vi "binary.vi"() -> ()   [LabVIEW 2020]
uses:
  <vilib>/Utility/error.llb/DialogType.ctl
panel:
  out "data":dbl[](array[numeric])
  out "Array":dbl[](array[numeric])
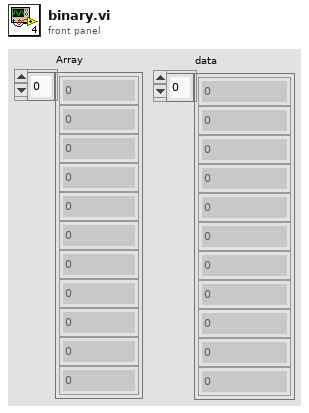
[diagram p1: front panel]
types:
  T1 = enum16{"open", "replace", "create", "open or create", "replace or create", "replace or create with confirmation"}
  T2 = typedef "DialogType.ctl" = u16
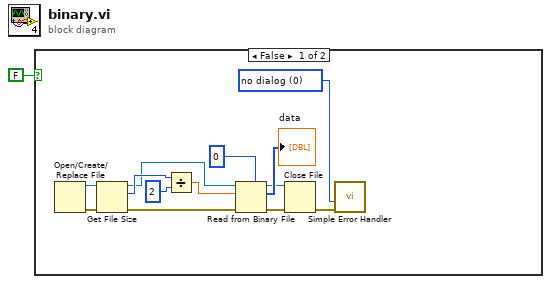
[diagram p0: block diagram]
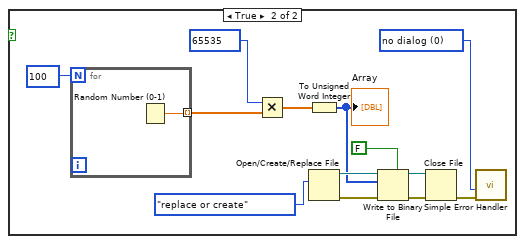
[diagram p2: hidden frame]
diagram:
  n1 = case shown="False" FALSE {
    frame False {
      w2 = T2 0 items=["no dialog", "OK message", "continue or stop message", "OK message + warnings", "continue/stop + warnings"] ("type of dialog (OK msg:1)")
      n2 = Open/Create/Replace File() -> (refnum out=w14:refnum<file>, error out=w13:errorcluster)  [unwired: 6 in, 1 out]
      n3 = Get File Size(file=w14, error in=w13) -> (refnum out=w10:refnum<file>, size (in bytes)=w12:i64, 0:w9:errorcluster)
      n4 = Divide(x=w12, y=i64 2) -> (x/y=w8:dbl)
      n5 = Read from Binary File(5:u16 0, 8:w9, 10:w8, 11:w10) -> (0:w4:errorcluster, 2:→"data":u16[], 3:w5:refnum<file>)  [unwired: 2 in, 1 out]
      n6 = Close File(refnum=w5, error in=w4) -> (error out=w3:errorcluster)  [unwired: 1 out]
      n7 = call <vilib>:"Simple Error Handler.vi"("type of dialog (OK msg:1)"=w2, "error in (no error)"=w3) -> ()  [unwired: 3 in, 5 out]
    }
    frame True {
      w18 = T2 0 items=["no dialog", "OK message", "continue or stop message", "OK message + warnings", "continue/stop + warnings"] ("type of dialog (OK msg:1)")
      n8 = for {
        N: 100 -> [_]
        tunnel: [w28] -> w23 mode=indexing
        n9 = Random Number (0-1)() -> (number: 0 to 1=w28:dbl)
      }
      n10 = Multiply(x=65535, y=w23) -> (x*y=w17:dbl[])
      n11 = To Unsigned Word Integer(number=w17) -> (unsigned 16bit integer=w15:u16[])
      "Array" <- w15
      n12 = Open/Create/Replace File(operation (0:open)=T1."replace or create") -> (refnum out=w25:refnum<file>, error out=w24:errorcluster)  [unwired: 5 in, 1 out]
      n13 = Write to Binary File(file (use dialog)=w25, data=w15, error in=w24, 5:FALSE ("prepend array or string size? (T)")) -> (refnum out=w20:refnum<file>, error out=w21:errorcluster)  [unwired: 2 in, 1 out]
      n14 = Close File(refnum=w20, error in=w21) -> (error out=w19:errorcluster)  [unwired: 1 out]
      n15 = call <vilib>:"Simple Error Handler.vi"("type of dialog (OK msg:1)"=w18, "error in (no error)"=w19) -> ()  [unwired: 3 in, 5 out]
    }
  }
